vi "SWERVE_DRIVE_ACT.vi"(6 "Pass_Through_Time":dbl=-1.0 format="%33.4f", 8 "error in":errorcluster) -> (0 "error out":errorcluster)   [LabVIEW 2023]
uses:
  <vilib>/Rock Robotics/WPI/ThirdParty/JAS_Junk/TrajLib/TypeDef/CHASSIS_SPEEDS.ctl
  <vilib>/Rock Robotics/WPI/ThirdParty/JAS_Junk/TrajLib/TypeDef/POSE2D.ctl
  <vilib>/Rock Robotics/WPI/ThirdParty/JAS_Junk/TrajLib/TypeDef/TRANSLATION2D.ctl
  <vilib>/Rock Robotics/WPI/ThirdParty/JAS_Junk/TrajLib/TypeDef/ROTATION2D.ctl
  <vilib>/Rock Robotics/WPI/ThirdParty/JAS_Junk/TrajLib/Enum/DCMOTOR_TYPES_ENUM.ctl
  36e0b83a-1a72-4a1b-a2b1-90e6be610630.vi
  <vilib>/Rock Robotics/WPI/ThirdParty/JAS_Junk/TrajLib/MathUtil_InputModulus.vi
  <vilib>/Rock Robotics/WPI/ThirdParty/JAS_Junk/TrajLib/Translation2d_Create.vi
  <vilib>/Rock Robotics/WPI/ThirdParty/JAS_Junk/TrajLib/PIDController_AtSetpoint.vi
  <vilib>/Rock Robotics/WPI/ThirdParty/JAS_Junk/TrajLib/PIDController_SetPIDF.vi
  <vilib>/Rock Robotics/WPI/ThirdParty/JAS_Junk/TrajLib/PIDController_SetDerivativeFilter.vi
  <vilib>/Rock Robotics/WPI/ThirdParty/JAS_Junk/TrajLib/PIDController_SetIntegratorRange.vi
  <vilib>/Rock Robotics/WPI/ThirdParty/JAS_Junk/TrajLib/PIDController_SetTolerancePandV.vi
  <vilib>/Rock Robotics/WPI/ThirdParty/JAS_Junk/TrajLib/PIDController_DisableContinousInput.vi
  <vilib>/Rock Robotics/WPI/ThirdParty/JAS_Junk/TrajLib/PIDController_EnableContinousInput.vi
  <vilib>/Rock Robotics/WPI/ThirdParty/JAS_Junk/TrajLib/PIDController_Reset.vi
  <vilib>/Rock Robotics/WPI/ThirdParty/JAS_Junk/TrajLib/PIDController_New.vi
  <vilib>/Rock Robotics/WPI/ThirdParty/JAS_Junk/TrajLib/PIDController_SetOutputLimits.vi
  <vilib>/Rock Robotics/WPI/ThirdParty/JAS_Junk/TrajLib/VI/PIDController_SetIntegratorZone.vi
  <vilib>/Rock Robotics/WPI/ThirdParty/JAS_Junk/TrajLib/Rotation2d_Minus.vi
  <vilib>/Rock Robotics/WPI/ThirdParty/JAS_Junk/TrajLib/Rotation2d_GetRadians.vi
  <vilib>/Rock Robotics/WPI/ThirdParty/JAS_Junk/TrajLib/Rotation2d_RotateBy.vi
  <vilib>/Rock Robotics/WPI/ThirdParty/JAS_Junk/TrajLib/ChassisSpeeds_FromFieldRelativeSpeeds.vi
  <vilib>/Rock Robotics/WPI/ThirdParty/JAS_Junk/TrajLib/PIDController_NewPeriod.vi
  <vilib>/Rock Robotics/WPI/ThirdParty/JAS_Junk/TrajLib/Rotation2d_CreateXY.vi
  <vilib>/Rock Robotics/WPI/ThirdParty/JAS_Junk/TrajLib/Rotation2d_GetCos.vi
  <vilib>/Rock Robotics/WPI/ThirdParty/JAS_Junk/TrajLib/Rotation2d_GetSin.vi
  <vilib>/Rock Robotics/SystemInterfaces/NetworkCommunication/NetComm_UsageReport_report.vi
  <vilib>/Rock Robotics/WPI/ThirdParty/JAS_Junk/TrajLib/Util_CalcDist.vi
  SWERVE_DRIVE_GLOBALS.vi
  Robot Global Data.vi
  <vilib>/Rock Robotics/Network Tables/NT Read Number.vi
  <vilib>/Rock Robotics/Network Tables/NT Write Numeric Array.vi
  <vilib>/Rock Robotics/WPI/ThirdParty/JAS_Junk/TrajLib/Globals/Util_LibraryGlobals.vi
  <vilib>/Rock Robotics/WPI/ThirdParty/JAS_Junk/TrajLib/PIDController_AdvCalculate_FF_Sp_Pv.vi
  <vilib>/Rock Robotics/Network Tables/NT Write Number.vi
  <vilib>/Rock Robotics/Network Tables/NT Write Boolean.vi
  <vilib>/Rock Robotics/WPI/ThirdParty/JAS_Junk/TrajLib/Trajectory_Library.lvlib
panel:
  out "Orientation PV":dbl
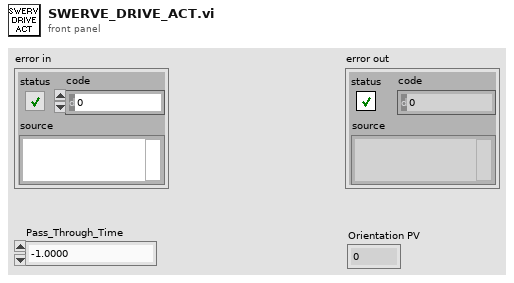
[diagram p1: front panel]
types:
  T1 = typedef "WPI_DriverStationRobotMode2.ctl" = enum16{"Autonomous Disabled", "Autonomous Enabled", "Teleop Disabled", "Teleop Enabled", "Disconnected", "Finish", "Test Disabled", "Test Enabled", "Emergency Stopped"}
  T2 = typedef "Trajectory_Library.lvlib/CHASSIS_SPEEDS.ctl" = cluster{"vX":dbl, "vY":dbl, "vOmega":dbl}
  T3 = typedef "Trajectory_Library.lvlib/POSE2D.ctl" = cluster{"TRANSLATION":T4, "ROTATION":T5}
  T4 = typedef "Trajectory_Library.lvlib/TRANSLATION2D.ctl" = cluster{"X":dbl, "Y":dbl}
  T5 = typedef "Trajectory_Library.lvlib/ROTATION2D.ctl" = cluster{"VALUE":dbl, "COS":dbl, "SIN":dbl}
  T6 = typedef "Trajectory_Library.lvlib/SWERVE_DRIVE_KINEMATICS.ctl" = cluster{"NumModules":i32, "InverseKinematics":T7, "ForwardKinematics":T7, "Modules":T4[], "PrevCoR":T4, "SavedModuleStates":T8[]}
  T7 = typedef "NI_Matrix.lvlib/RealMatrix.ctl" = dbl[][]
  T8 = typedef "Trajectory_Library.lvlib/SWERVE_DRIVE_MODULE_STATE.ctl" = cluster{"Speed":dbl, "Angle":T5}
  T9 = typedef "Trajectory_Library.lvlib/PID_ADV_LIMITS.ctl" = cluster{"MaxInput":dbl, "MinInput":dbl, "Continuous":bool, "MaxOutput":dbl, "MinOutput":dbl}
  T10 = typedef "Trajectory_Library.lvlib/PID_ADV_TUNING.ctl" = cluster{"Kf":dbl, "Kp":dbl, "Ki":dbl, "Kd":dbl, "MaximumIntegral":dbl, "MinimumIntegral":dbl, "Filter Derivative":bool, "IntegralZone":dbl}
  T11 = typedef "Trajectory_Library.lvlib/TWIST2D.ctl" = cluster{"dX":dbl, "dY":dbl, "dTHETA":dbl}
  T12 = typedef "Trajectory_Library.lvlib/DCMOTOR_TYPES_ENUM.ctl" = enum16{"CIM", "AndyMark 9015", "Andy Mark RS 775 125", "Bag", "BaneBots RS 550", "BaneBots RS 775", "Falcon 500", "Mini CIM", "NEO", "NEO 550", "Romi BuiltIn", "Vex 775 Pro", "Snow Blower AM 2235A", "Bosch Seat AM 3493", "Falcon 500 FOC", "Kraken X60", "Kraken X60 FOC", "NEO Vortex"}
  T13 = cluster{"Motor Name":string, "MC type":enum16{"Talon FX, P5", "Talon FX, P6", "SPARK MAX"}, "Motor Type":T12, "Gear Ratio":dbl}
  T14 = enum16{"Talon FX, P5", "Talon FX, P6", "SPARK MAX"}
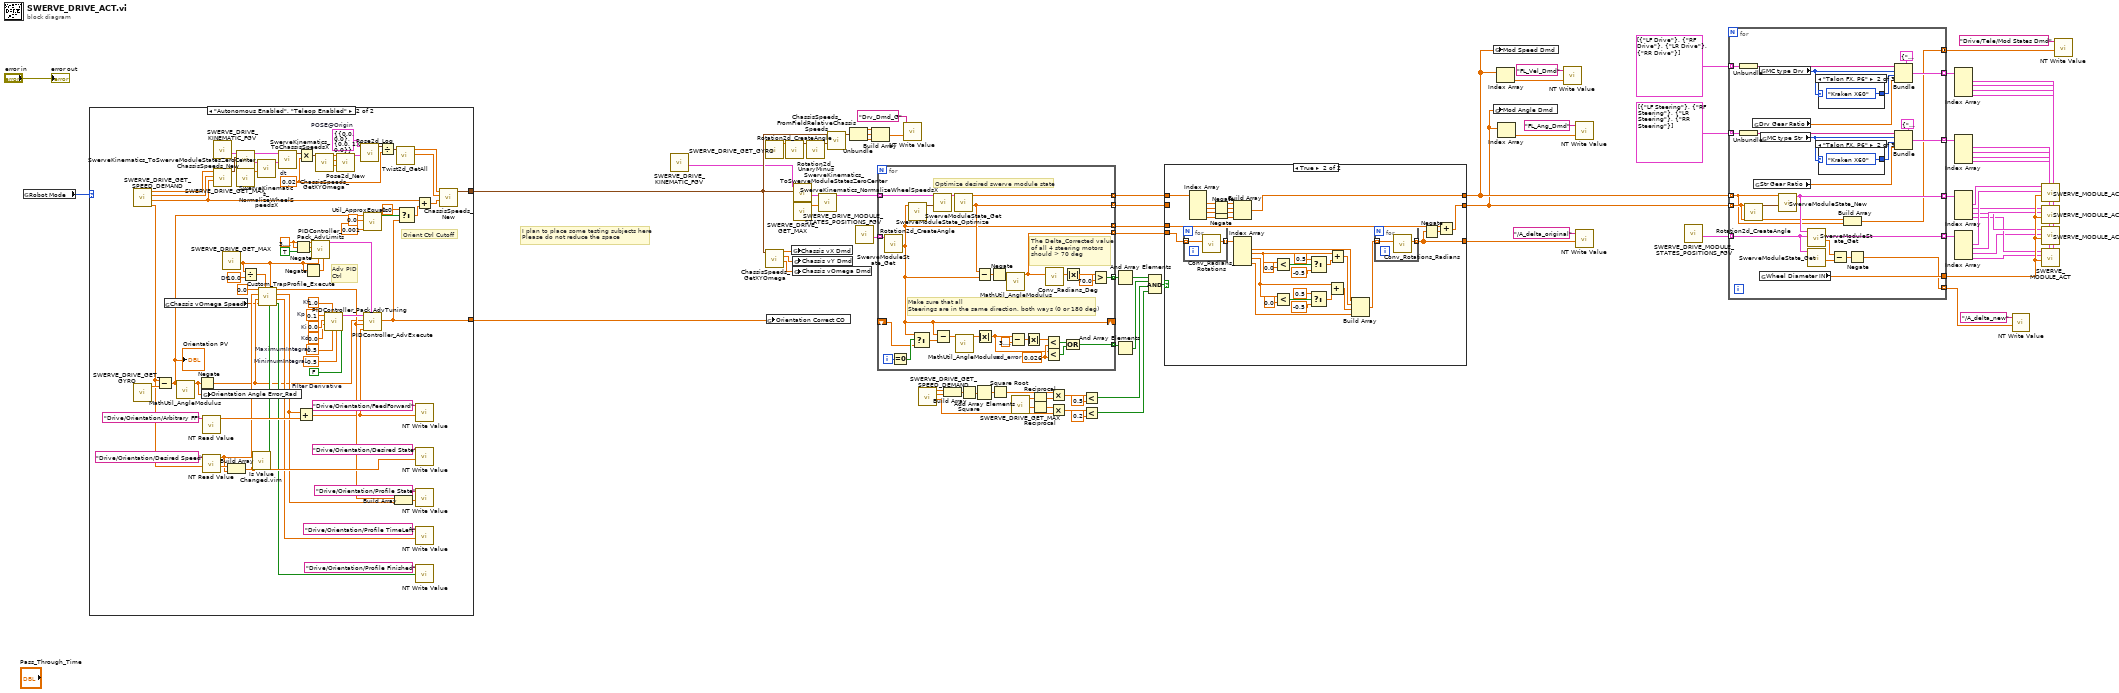
[diagram p0: block diagram]
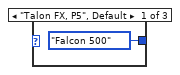
[diagram p2: hidden frame]
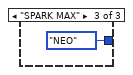
[diagram p3: hidden frame]
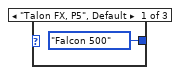
[diagram p4: hidden frame]
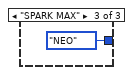
[diagram p5: hidden frame]
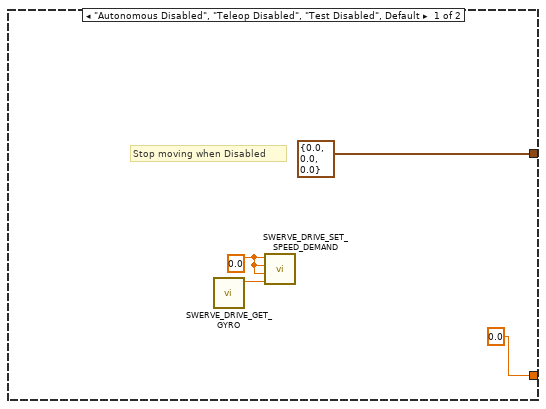
[diagram p6: hidden frame]
diagram:
  # "I plan to place some testing subjects here\nPlease do not reduce the space"
  n1 = global read "Robot Global Data.vi" "Robot Mode"() -> (w57:T1)
  n2 = case shown="\"Autonomous Enabled\", \"Teleop Enabled\"" w57 {
    tunnel: [T2 {"vX"=0.0, "vY"=0.0, "vOmega"=0.0} ("CHASSIS") w156] -> w83
    tunnel: [0.0 ("CO-ControlOutput") w89] -> w67
    frame "Autonomous Disabled", "Teleop Disabled", "Test Disabled", Default {
      w86 = 0.0 ("Drv X Vel Dmd")
      # "Stop moving when Disabled"
      n3 = call "SWERVE_DRIVE_GET_GYRO.vi"() -> ("Gyro Heading Radians"=w85:dbl)  [unwired: 11 in]
      n4 = call "SWERVE_DRIVE_SET_SPEED_DEMAND.vi"("Drv Rotation Orentation Dmd"=w85, "Drv Angular Vel Dmd"=w86, "Drv Y Vel Dmd"=w86, "Drv X Vel Dmd"=w86) -> ()  [unwired: 8 in]
    }
    frame "Autonomous Enabled", "Teleop Enabled" {
      w116 = 0.1  # Kp
      w115 = 0.0  # Ki
      w114 = 0.0  # Kd
      w132 = T3 {"TRANSLATION"={"X"=0.0, "Y"=0.0}, "ROTATION"={"VALUE"=0.0, "COS"=1.0, "SIN"=0.0}}  # POSE@Origin
      w131 = 0.02  # dt
      w146 = 10.0  # Dt
      w145 = 1.0  # Kf
      w152 = 0.5  # MaximumIntegral
      w151 = -0.5  # MinimumIntegral
      w150 = FALSE  # Filter Derivative
      w153 = 3.141592653589793
      # "Orient Ctrl Cutoff"
      # "Adv PID\nCtrl"
      n5 = call "SWERVE_DRIVE_GET_SPEED_DEMAND.vi"() -> ("Drv Rotation Orentation Dmd"=w109:dbl, "Drv Angular Vel Dmd"=w97:dbl, "Drv Y Vel Dmd"=w126:dbl, "Drv X Vel Dmd"=w128:dbl)  [unwired: 7 in, 1 out]
      n6 = call "SWERVE_DRIVE_GET_GYRO.vi"() -> ("Gyro Heading Radians"=w117:dbl)  [unwired: 11 in]
      n7 = Subtract(x=w109, y=w117) -> (x-y=w94:dbl)
      "Orientation PV" <- w94
      n8 = global read "SWERVE_DRIVE_GLOBALS.vi" "Chassis vOmega Speed"() -> (w96:dbl)
      n9 = call <vilib>:"MathUtil_AngleModulus.vi"("InputAngle"=w94) -> ("ModulsAngle"=w123:dbl)  [unwired: 10 in]
      n10 = Negate(x=w123) -> (-x=w98:dbl)
      n11 = global write "SWERVE_DRIVE_GLOBALS.vi" "Orientation Angle Error_Rad"(w123) -> ()
      n12 = call-poly <vilib>:"NT Read Value.vi"("name"="Drive/Orientation/Arbitrary FF") -> ("value"=w112:dbl)  [unwired: 8 in, 2 out]
      n13 = call-poly <vilib>:"NT Read Value.vi"("name"="Drive/Orientation/Desired Speed") -> ("value"=w106:dbl)  [unwired: 8 in, 2 out]
      n14 = call "SWERVE_DRIVE_KINEMATIC_FGV.vi"() -> ("out SWERVE_DRIVE_KINEMATICS"=w144:T6)  [unwired: 11 in]
      n15 = call <vilib>:"ChassisSpeeds_New.vi"("vAngular"=w97, "vY"=w126, "vX"=w128) -> ("CHASSIS"=w141:T2)  [unwired: 8 in]
      n16 = call "SWERVE_DRIVE_GET_MAX.vi"() -> ("Max Rotational Vel (Rad/Sec)"=w104:dbl)  [unwired: 10 in, 1 out]
      n17 = Build Array(w109, w106) -> (w108:dbl[])
      n18 = call <vilib>:"SwerveKinematics_ToSwerveModuleStatesZeroCenter.vi"("ChassisSpeeds"=w141, "in SWERVE_DRIVE_KINEMATICS"=w144) -> ("ModuleStates"=w143:T8[], "out SWERVE_DRIVE_KINEMATICS"=w140:T6)  [unwired: 8 in]
      n19 = call "SWERVE_DRIVE_GET_MAX.vi"() -> ("Max Wheel Vel (Meter/Sec)"=w142:dbl)  [unwired: 10 in, 1 out]
      n20 = Divide(x=w104, y=w146) -> (x/y=w103:dbl)
      n21 = call "Is Value Changed.vim"("value"=w108) -> ("changed or first call?"=w105:bool)
      n22 = call <vilib>:"SwerveKinematics_NormalizeWheelSpeedsX.vi"("AttainableMaxSpeed"=w142, "in WheelStates"=w143) -> ("out WheelStates"=w139:T8[])  [unwired: 9 in]
      n23 = call "Custom_TrapProfile_Execute.vi"("Initialize"=w105, "Max Speed"=w104, "Max Accel"=w103, "CurrentVelocity"=w96, "CurrentPosition"=w98, "GoalVelocity"=w106, "GoalPosition"=0.0) -> ("TimeFinished"=w99:bool, "EstTimeLeft"=w100:dbl, "VelocityDmd"=w101:dbl, "PositionDmd"=w102:dbl)  [unwired: 1 in]
      n24 = call <vilib>:"SwerveKinematics_ToChassisSpeedsX.vi"("WheelStates"=w139, "in SWERVE_DRIVE_KINEMATICS"=w140) -> ("Chassis Speed"=w138:T2)  [unwired: 9 in]
      n25 = Negate(x=w153) -> (-x=w154:dbl)
      n26 = Add(x=w101, y=w112) -> (x+y=w95:dbl)
      n27 = Multiply(x=w138, y=w131) -> (x*y=w137:T2)
      n28 = Negate(x=w104) -> (-x=w147:dbl)
      n29 = call <vilib>:"PIDController_Pack_AdvLimits.vi"("MinOutput"=w147, "MaxOutput"=w104, "Continuous"=TRUE, "MinInput"=w154, "MaxInput"=w153) -> ("Adv PID Limits"=w148:T9)  [unwired: 6 in]
      n30 = call <vilib>:"ChassisSpeeds_GetXYOmega.vi"("CHASSIS"=w137) -> ("vAngular"=w134:dbl, "vY"=w135:dbl, "vX"=w136:dbl)  [unwired: 8 in]
      n31 = call <vilib>:"PIDController_Pack_AdvTuning.vi"("Filter Derivative"=w150, "MinimumIntegral"=w151, "MaximumIntegral"=w152, "Kf"=w145, "Kd"=w114, "Ki"=w115, "Kp"=w116) -> ("Adv PID Tuning"=w149:T10)  [unwired: 4 in]
      n32 = call <vilib>:"Pose2d_New.vi"("Heading"=w134, "Y"=w135, "X"=w136) -> ("out POSe"=w133:T3)  [unwired: 8 in]
      n33 = call <vilib>:"Pose2d_Log.vi"("end POSE"=w133, "in POSE"=w132) -> ("out TWIST"=w130:T11)  [unwired: 9 in]
      n34 = call <vilib>:"Util_ApproxEquals.vi"("Tolerance"=0.001, "Value 2"=0.0, "Value 1"=w94) -> ("ApproxEquals"=w91:bool)  [unwired: 8 in]
      n35 = call <vilib>:"PIDController_AdvExecute.vi"("Adv PID Limits"=w148, "FF-FeedForward"=w95, "SP-SetPoint"=w102, "PV-Measurement"=w98, "Adv PID Tuning"=w149) -> ("CO-ControlOutput"=w89:dbl)  [unwired: 4 in, 2 out]
      n36 = Divide(x=w130, y=w131) -> (x/y=w129:T11)
      n37 = Build Array(w102, w101) -> (w119:dbl[])
      n38 = call <vilib>:"Twist2d_GetAll.vi"("TWIST"=w129) -> ("dY"=w125:dbl, "dX"=w127:dbl)  [unwired: 8 in, 1 out]
      n39 = Select(t=0.0, s=w91, f=w89) -> (s? t:f=w88:dbl)
      n40 = Add(x=w97, y=w88) -> (x+y=w118:dbl)
      n41 = call-poly <vilib>:"NT Write Value.vi"("value"=w95, "name"="Drive/Orientation/FeedForward") -> ()  [unwired: 9 in, 1 out]
      n42 = call-poly <vilib>:"NT Write Value.vi"("value"=w108, "name"="Drive/Orientation/Desired State") -> ()  [unwired: 9 in, 1 out]
      n43 = call-poly <vilib>:"NT Write Value.vi"("value"=w119, "name"="Drive/Orientation/Profile State") -> ()  [unwired: 9 in, 1 out]
      n44 = call-poly <vilib>:"NT Write Value.vi"("value"=w100, "name"="Drive/Orientation/Profile TimeLeft") -> ()  [unwired: 9 in, 1 out]
      n45 = call-poly <vilib>:"NT Write Value.vi"("value"=w99, "name"="Drive/Orientation/Profile Finished") -> ()  [unwired: 9 in, 1 out]
      n46 = call <vilib>:"ChassisSpeeds_New.vi"("vAngular"=w118, "vY"=w125, "vX"=w127) -> ("CHASSIS"=w156:T2)  [unwired: 8 in]
    }
  }
  n47 = call "SWERVE_DRIVE_KINEMATIC_FGV.vi"() -> ("out SWERVE_DRIVE_KINEMATICS"=w81:T6)  [unwired: 11 in]
  n48 = call "SWERVE_DRIVE_GET_GYRO.vi"() -> ("Gyro Heading Radians"=w72:dbl)  [unwired: 11 in]
  n49 = call <vilib>:"ChassisSpeeds_GetXYOmega.vi"("CHASSIS"=w83) -> ("vAngular"=w60:dbl, "vY"=w59:dbl, "vX"=w58:dbl)  [unwired: 8 in]
  n50 = global write "SWERVE_DRIVE_GLOBALS.vi" "Orientation Correct CO"(w67) -> ()
  n51 = call <vilib>:"Rotation2d_CreateAngle.vi"("Angle"=w72) -> ("ROTATION"=w74:T5)  [unwired: 10 in]
  n52 = global write "SWERVE_DRIVE_GLOBALS.vi" "Chassis vX Dmd"(w58) -> ()
  n53 = global write "SWERVE_DRIVE_GLOBALS.vi" "Chassis vY Dmd"(w59) -> ()
  n54 = global write "SWERVE_DRIVE_GLOBALS.vi" "Chassis vOmega Dmd"(w60) -> ()
  n55 = call <vilib>:"SwerveKinematics_ToSwerveModuleStatesZeroCenter.vi"("ChassisSpeeds"=w83, "in SWERVE_DRIVE_KINEMATICS"=w81) -> ("ModuleStates"=w82:T8[])  [unwired: 8 in, 1 out]
  n56 = call "SWERVE_DRIVE_GET_MAX.vi"() -> ("Max Wheel Vel (Meter/Sec)"=w36:dbl)  [unwired: 10 in, 1 out]
  n57 = call <vilib>:"Rotation2d_UnaryMinus.vi"("in ROTATION"=w74) -> ("out ROTATION"=w73:T5)  [unwired: 10 in]
  n58 = call <vilib>:"SwerveKinematics_NormalizeWheelSpeedsX.vi"("AttainableMaxSpeed"=w36, "in WheelStates"=w82) -> ("out WheelStates"=w35:T8[])  [unwired: 9 in]
  n59 = call <vilib>:"ChassisSpeeds_FromFieldRelativeChassisSpeeds.vi"("RobotAngle"=w73, "FieldRelChassisSPeeds"=w83) -> ("CHASSIS"=w75:T2)  [unwired: 9 in]
  n60 = Unbundle(w75) -> ("vX"=w76:dbl, "vY"=w77:dbl, "vOmega"=w78:dbl)
  n61 = call "SWERVE_DRIVE_MODULE_STATES_POSITIONS_FGV.vi"() -> ("out Current Module States"=w34:T8[])  [unwired: 10 in, 1 out]
  n62 = Build Array(w76, w77, w78) -> (w79:dbl[])
  n63 = for {
    tunnel: w35 -> [w184] mode=indexing
    tunnel: w34 -> [w174] mode=indexing
    tunnel: [w179] -> w39 mode=indexing
    tunnel: [w181] -> w40 mode=indexing
    tunnel: [w175] -> w37 mode=indexing
    tunnel: [w157] -> w41 mode=indexing
    shift-right: [w159] -> _
    shift-left: _ -> [w172]
    tunnel: [w161] -> w62 mode=indexing
    tunnel: [w159] -> w66 mode=indexing
    i -> [w160]
    w166 = 0.026  # rad_error
    # "Make sure that all\nSteerings are in the same direction, both ways (0 or 180 deg)"
    # "The Delta_Corrected value of all 4 steering motors should > 70 deg"
    # "Optimize desired swerve module state"
    n64 = call <vilib>:"SwerveModuleState_Get.vi"("Desired State"=w174) -> ("Angle RADIANS"=w159:dbl)  [unwired: 9 in, 1 out]
    n65 = Equal To 0?(x=w160) -> (x = 0?=w173:bool)
    n66 = call <vilib>:"Rotation2d_CreateAngle.vi"("Angle"=w159) -> ("ROTATION"=w183:T5)  [unwired: 10 in]
    n67 = Select(t=w159, s=w173, f=w172) -> (s? t:f=w171:dbl)
    n68 = call <vilib>:"SwerveModuleState_Optimize.vi"("CurrentAngle"=w183, "Desired State"=w184) -> ("out SWERVE_DRIVE_MODULE_STATE"=w182:T8)  [unwired: 9 in]
    n69 = Subtract(x=w159, y=w171) -> (x-y=w167:dbl)
    n70 = call <vilib>:"SwerveModuleState_Get.vi"("Desired State"=w182) -> ("Angle RADIANS"=w181:dbl, "Speed M/S"=w179:dbl)  [unwired: 9 in]
    n71 = call <vilib>:"MathUtil_AngleModulus.vi"("InputAngle"=w167) -> ("ModulsAngle"=w170:dbl)  [unwired: 10 in]
    n72 = Subtract(x=w181, y=w159) -> (x-y=w180:dbl)
    n73 = Absolute Value(x=w170) -> (abs(x)=w164:dbl)
    n74 = Negate(x=w180) -> (-x=w158:dbl)
    n75 = call <vilib>:"MathUtil_AngleModulus.vi"("InputAngle"=w158) -> ("ModulsAngle"=w157:dbl)  [unwired: 10 in]
    n76 = Subtract(x=w164, y=3.141592653589793) -> (x-y=w169:dbl)
    n77 = Absolute Value(x=w169) -> (abs(x)=w165:dbl)
    n78 = Less?(x=w165, y=w166) -> (x < y?=w163:bool)
    n79 = Less?(x=w164, y=w166) -> (x < y?=w162:bool)
    n80 = call <vilib>:"Conv_Radians_Deg.vi"("Radians"=w157) -> ("Degrees"=w178:dbl)  [unwired: 10 in]
    n81 = Absolute Value(x=w178) -> (abs(x)=w177:dbl)
    n82 = Compound Arithmetic op=OR(w163, w162) -> (w161:bool)
    n83 = Greater?(x=w177, y=70.0) -> (0:w175:bool)
  }
  n84 = call-poly <vilib>:"NT Write Value.vi"("value"=w79, "name"="Drv_Dmd_G") -> ()  [unwired: 9 in, 1 out]
  n85 = call "SWERVE_DRIVE_GET_SPEED_DEMAND.vi"() -> ("Drv Angular Vel Dmd"=w52:dbl, "Drv Y Vel Dmd"=w43:dbl, "Drv X Vel Dmd"=w42:dbl)  [unwired: 7 in, 2 out]
  n86 = Build Array(w42, w43) -> (w46:dbl[])
  n87 = Square(x=w46) -> (x^2=w47:dbl[])
  n88 = Add Array Elements(numeric array=w47) -> (sum=w48:dbl)
  n89 = Square Root(x=w48) -> (sqrt(x)=w50:dbl)
  n90 = call "SWERVE_DRIVE_GET_MAX.vi"() -> ("Max Rotational Vel (Rad/Sec)"=w45:dbl, "Max Wheel Vel (Meter/Sec)"=w44:dbl)  [unwired: 10 in]
  n91 = Reciprocal(x=w44) -> (1/x=w49:dbl)
  n92 = Reciprocal(x=w45) -> (1/x=w51:dbl)
  n93 = Multiply(x=w50, y=w49) -> (x*y=w54:dbl)
  n94 = Multiply(x=w51, y=w52) -> (x*y=w56:dbl)
  n95 = Less?(x=w54, y=0.5) -> (x < y?=w64:bool)
  n96 = Less?(x=w56, y=0.2) -> (x < y?=w65:bool)
  n97 = And Array Elements(Boolean array=w37) -> (logical AND=w61:bool)
  n98 = And Array Elements(Boolean array=w62) -> (logical AND=w63:bool)
  n99 = Compound Arithmetic op=AND(w61, w63, w64, w65) -> (w38:bool)
  n100 = case shown="True" w38 {
    tunnel: w39 -> [w187 w196]
    tunnel: w40 -> [w186 _]
    tunnel: w41 -> [w185 w200]
    tunnel: [w187 w189] -> w30
    tunnel: [w186 w217] -> w29
    tunnel: [w185 w197] -> w5
    tunnel: w66 -> [_ w188]
    frame False {
    }
    frame True {
      n101 = for {
        tunnel: w200 -> [w222] mode=indexing
        tunnel: [w221] -> w199 mode=indexing
        n102 = call <vilib>:"Conv_Radians_Rotations.vi"("Radians"=w222) -> ("Rotations"=w221:dbl)  [unwired: 10 in]
      }
      n103 = Index Array(array=w196) -> (element #1=w193:dbl, element #2=w195:dbl, element #3=w194:dbl, element #4=w190:dbl)  [unwired: 4 in]
      n104 = Negate(x=w195) -> (-x=w192:dbl)
      n105 = Negate(x=w194) -> (-x=w191:dbl)
      n106 = Build Array(w193, w192, w191, w190) -> (w189:dbl[])
      n107 = Index Array(array=w199) -> (element #1=w206:dbl, element #2=w207:dbl, element #3=w201:dbl, element #4=w203:dbl)  [unwired: 4 in]
      n108 = Less?(x=w207, y=0.0) -> (x < y?=w214:bool)
      n109 = Less?(x=w201, y=0.0) -> (x < y?=w209:bool)
      n110 = Select(t=0.5, s=w214, f=-0.5) -> (s? t:f=w208:dbl)
      n111 = Select(t=0.5, s=w209, f=-0.5) -> (s? t:f=w202:dbl)
      n112 = Add(x=w201, y=w202) -> (x+y=w204:dbl)
      n113 = Add(x=w207, y=w208) -> (x+y=w205:dbl)
      n114 = Build Array(w206, w205, w204, w203) -> (w198:dbl[])
      n115 = for {
        tunnel: w198 -> [w220] mode=indexing
        tunnel: [w219] -> w197 mode=indexing
        n116 = call <vilib>:"Conv_Rotations_Radians.vi"("Rotations"=w220) -> ("Radians"=w219:dbl)  [unwired: 10 in]
      }
      n117 = Negate(x=w197) -> (-x=w218:dbl[])
      n118 = Add(x=w188, y=w218) -> (x+y=w217:dbl[])
    }
  }
  n119 = global write "SWERVE_DRIVE_GLOBALS.vi" "Mod Speed Dmd"(w30) -> ()
  n120 = global write "SWERVE_DRIVE_GLOBALS.vi" "Mod Angle Dmd"(w29) -> ()
  n121 = Index Array(array=w30) -> (element=w68:dbl)  [unwired: 1 in]
  n122 = Index Array(array=w29) -> (element=w70:dbl)  [unwired: 1 in]
  n123 = call-poly <vilib>:"NT Write Value.vi"("value"=w68, "name"="FL_Vel_Dmd") -> ()  [unwired: 9 in, 1 out]
  n124 = call-poly <vilib>:"NT Write Value.vi"("value"=w70, "name"="FL_Ang_Dmd") -> ()  [unwired: 9 in, 1 out]
  n125 = call-poly <vilib>:"NT Write Value.vi"("value"=w5, "name"="/A_delta_original") -> ()  [unwired: 9 in, 1 out]
  n126 = call "SWERVE_DRIVE_MODULE_STATES_POSITIONS_FGV.vi"() -> ("out Current Module States"=w28:T8[])  [unwired: 10 in, 1 out]
  n127 = for {
    tunnel: cluster{string}[] [{"LF Drive"}, {"RF Drive"}, {"LR Drive"}, {"RR Drive"}] ("Steering ref") -> [w247] mode=indexing
    tunnel: cluster{string}[] [{"LF Steering"}, {"RF Steering"}, {"LR Steering"}, {"RR Steering"}] ("Steering ref") -> [w246] mode=indexing
    tunnel: [w238] -> w26 mode=indexing
    tunnel: [w237] -> w27 mode=indexing
    tunnel: [w236] -> w19
    tunnel: w30 -> [w227] mode=indexing
    tunnel: w29 -> [w228] mode=indexing
    tunnel: w28 -> [w232] mode=indexing
    tunnel: [w232] -> w25 mode=indexing
    tunnel: [w231] -> w24 mode=indexing
    tunnel: [w230] -> w3 mode=indexing
    tunnel: [w229] -> w1 mode=concatenating
    n128 = Unbundle(w247) -> (w241:string)
    n129 = Unbundle(w246) -> (w240:string)
    n130 = call <vilib>:"Rotation2d_CreateAngle.vi"("Angle"=w228) -> ("ROTATION"=w239:T5)  [unwired: 10 in]
    n131 = global read "SWERVE_DRIVE_GLOBALS.vi" "Drv Gear Ratio"() -> (w244:dbl)
    n132 = global read "SWERVE_DRIVE_GLOBALS.vi" "Str Gear Ratio"() -> (w245:dbl)
    n133 = global read "SWERVE_DRIVE_GLOBALS.vi" "MC type Drv"() -> (w226:T14)
    n134 = global read "SWERVE_DRIVE_GLOBALS.vi" "Wheel Diameter IN"() -> (w236:dbl)
    n135 = global read "SWERVE_DRIVE_GLOBALS.vi" "MC type Str"() -> (w225:T14)
    n136 = call <vilib>:"SwerveModuleState_New.vi"("ROTATION"=w239, "Speed"=w227) -> ("SWERVE_DRIVE_MODULE_STATE"=w231:T8)  [unwired: 9 in]
    n137 = call <vilib>:"SwerveModuleState_Get.vi"("Desired State"=w231) -> ("Angle RADIANS"=w233:dbl)  [unwired: 9 in, 1 out]
    n138 = call <vilib>:"SwerveModuleState_Get.vi"("Desired State"=w232) -> ("Angle RADIANS"=w235:dbl)  [unwired: 9 in, 1 out]
    n139 = case shown="\"Talon FX, P6\"" w226 {
      tunnel: [DCMOTOR_TYPES_ENUM."Falcon 500" ("DCMOTOR_TYPES") DCMOTOR_TYPES_ENUM."Kraken X60" ("DCMOTOR_TYPES") DCMOTOR_TYPES_ENUM."NEO" ("DCMOTOR_TYPES")] -> w224
      frame "Talon FX, P5", Default {
      }
      frame "Talon FX, P6" {
      }
      frame "SPARK MAX" {
      }
    }
    n140 = case shown="\"Talon FX, P6\"" w225 {
      tunnel: [DCMOTOR_TYPES_ENUM."Falcon 500" ("DCMOTOR_TYPES") DCMOTOR_TYPES_ENUM."Kraken X60" ("DCMOTOR_TYPES") DCMOTOR_TYPES_ENUM."NEO" ("DCMOTOR_TYPES")] -> w223
      frame "Talon FX, P5", Default {
      }
      frame "Talon FX, P6" {
      }
      frame "SPARK MAX" {
      }
    }
    n141 = Subtract(x=w233, y=w235) -> (x-y=w234:dbl)
    n142 = Build Array(w228, w227) -> (w229:dbl[])
    n143 = Negate(x=w234) -> (-x=w230:dbl)
    n144 = Bundle(cluster=T13 {"Motor Name"="LF Drive", "MC type"=enum."Talon FX, P5", "Motor Type"=enum."NEO", "Gear Ratio"=0.0} ("Drive Motor Info"), "Motor Name"=w241, "MC type"=w226, "Motor Type"=w224, "Gear Ratio"=w244) -> (w237:T13)
    n145 = Bundle(cluster=T13 {"Motor Name"="LF Steering", "MC type"=enum."Talon FX, P5", "Motor Type"=enum."NEO", "Gear Ratio"=0.0} ("Steering Motor Info"), "Motor Name"=w240, "MC type"=w225, "Motor Type"=w223, "Gear Ratio"=w245) -> (w238:T13)
  }
  n146 = Index Array(array=w27) -> (element #1=w22:T13, element #2=w15:T13, element #3=w14:T13, element #4=w13:T13)  [unwired: 4 in]
  n147 = Index Array(array=w26) -> (element #1=w23:T13, element #2=w12:T13, element #3=w11:T13, element #4=w10:T13)  [unwired: 4 in]
  n148 = Index Array(array=w24) -> (element #1=w21:T8, element #2=w18:T8, element #3=w16:T8, element #4=w9:T8)  [unwired: 4 in]
  n149 = Index Array(array=w25) -> (element #1=w20:T8, element #2=w17:T8, element #3=w8:T8, element #4=w7:T8)  [unwired: 4 in]
  n150 = call-poly <vilib>:"NT Write Value.vi"("value"=w3, "name"="/A_delta_new") -> ()  [unwired: 9 in, 1 out]
  n151 = call "SWERVE_MODULE_ACT.vi"("Drive Motor Info"=w22, "Steering Motor Info"=w23, "Wheel Diameter IN"=w19, "Swerve State"=w20, "Swerve Dmd"=w21) -> ()  [unwired: 7 in]
  n152 = call "SWERVE_MODULE_ACT.vi"("Drive Motor Info"=w15, "Steering Motor Info"=w12, "Wheel Diameter IN"=w19, "Swerve State"=w17, "Swerve Dmd"=w18) -> ()  [unwired: 7 in]
  n153 = call "SWERVE_MODULE_ACT.vi"("Drive Motor Info"=w14, "Steering Motor Info"=w11, "Wheel Diameter IN"=w19, "Swerve State"=w8, "Swerve Dmd"=w16) -> ()  [unwired: 7 in]
  n154 = call "SWERVE_MODULE_ACT.vi"("Drive Motor Info"=w13, "Steering Motor Info"=w10, "Wheel Diameter IN"=w19, "Swerve State"=w7, "Swerve Dmd"=w9) -> ()  [unwired: 7 in]
  n155 = call-poly <vilib>:"NT Write Value.vi"("value"=w1, "name"="Drive/Tele/Mod States Dmd") -> ()  [unwired: 9 in, 1 out]
  "error out" <- "error in"
